vi "Destroy.vi"(8 "error in (no error)":errorcluster, 9 "force destroy? (F)":bool, 11 "Future in":refnum<class "Future.lvclass">) -> (0 "error out":errorcluster)   [LabVIEW 2017, in "Promise Future.lvlib" / "Future.lvclass"]
uses:
  Future.lvclass
  Future.lvclass/Future.ctl
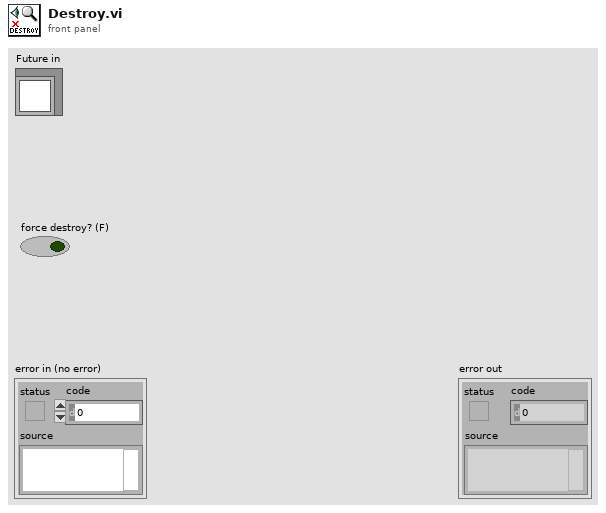
[diagram p1: front panel]
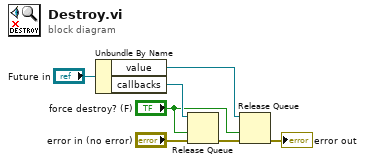
[diagram p0: block diagram]
diagram:
  n1 = Unbundle By Name("Future in") -> ("value"=w6:refnum<queue>, "callbacks"=w4:refnum<queue>)
  n2 = Release Queue(queue=w4, force destroy? (F)="force destroy? (F)", error in (no error)="error in (no error)") -> (error out=w1:errorcluster)  [unwired: 2 out]
  n3 = Release Queue(queue=w6, force destroy? (F)="force destroy? (F)", error in (no error)=w1) -> (error out=→"error out":errorcluster)  [unwired: 2 out]
